vi "Get Varietal.vi"(8 "error in (no error)":errorcluster, 11 "Leaf in":refnum<class "Leaf.lvclass">) -> (0 "error out":errorcluster, 2 "Varietal":string, 3 "Leaf out":refnum<class "Leaf.lvclass">)   [LabVIEW 2021, in "Bananas.lvlib" / "Leaf.lvclass"]
uses:
  Leaf.lvclass
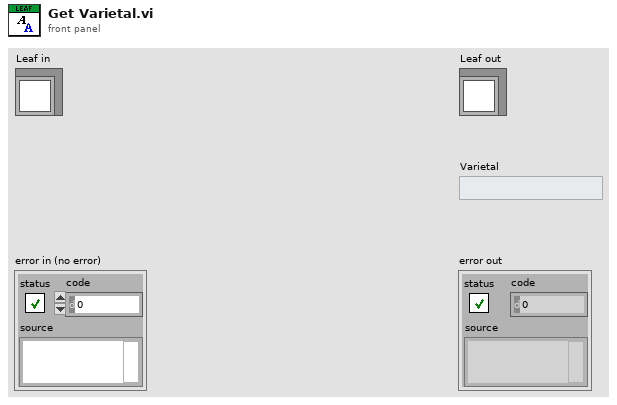
[diagram p1: front panel]
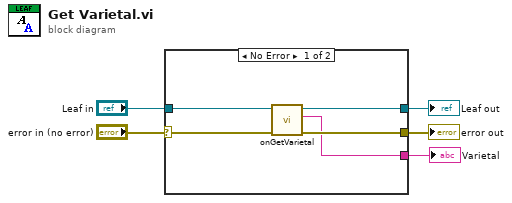
[diagram p0: block diagram]
diagram:
  n1 = case shown="No Error" "error in (no error)" {
    selector: "error in (no error)" -> [w8 w12]
    tunnel: [w7 w12] -> w4
    tunnel: [w10 w11] -> w2
    tunnel: "Leaf in" -> [w9 w11]
    tunnel: [w6 _] -> w1
    frame No Error {
      n2 = call-dynamic "onGetVarietal.vi"("error in (no error)"=w8, "Leaf in"=w9) -> ("error out"=w7:errorcluster, "Varietal"=w6:string, "Leaf out"=w10:refnum<class "Leaf.lvclass">)  [unwired: 7 in]
    }
    frame Error {
    }
  }
  "error out" <- w4
  "Leaf out" <- w2
  "Varietal" <- w1
